vi "ROI entry-Handle ROI change.vi"(7 "Selected ROI":i32[](array[numeric]), 8 "error in (no error)":errorcluster, 9 "Offsets cluster":T1, 11 "ROI management":T2) -> (0 "error out":errorcluster, 2 "No ROI":bool, 3 "Number of ROI":i32)   [LabVIEW 2020]
uses:
  Typedefs/ROI management FG states.ctl
  Typedefs/Offsets cluster.ctl
  ROI Entry screen/Typedefs/Redraw ROI.ctl
  ROI Entry screen/Typedefs/FGV ROI Time Ops.ctl
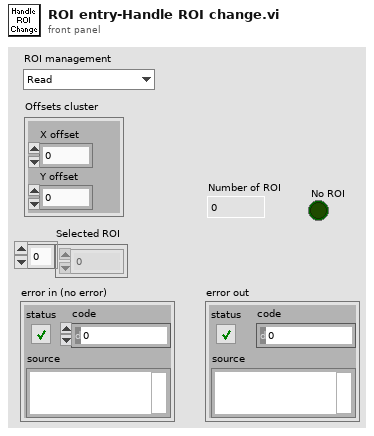
[diagram p1: front panel]
types:
  T1 = typedef "Offsets cluster.ctl" = cluster{"X offset":i8, "Y offset":i8}
  T2 = typedef "ROI management FG states.ctl" = enum16{"Read", "Write", "Write-from dataset", "Clear Last", "Clear All", "Delete ROI", "Update ROIs time", "Reload last ROI set", "Modify ROI Parameters", "Offset all ROI", "Offset visible ROI", "Modify Dwell Time", "Modify Laser Power"}
  T3 = typedef "FGV ROI Time Ops.ctl" = enum16{"Read", "Write Cycle Time", "Write Cycle Rate"}
  T4 = typedef "Redraw ROI.ctl" = enum16{"Redraw All", "Redraw Deselected", "Draw Last", "Redraw Selected"}
  T5 = typedef "ROI parameters data type.ctl" = cluster{"ROI index":dbl, "ROI ID":dbl, "ROI Time (ns)":dbl, "Pixels in ROI":dbl, "X start":dbl, "Y start":dbl, "Z start":dbl, "X stop":dbl, "Y stop":dbl, "Z stop":dbl, "Angle (deg)":dbl, "Composite ID":dbl, "Number of lines":dbl, "Frame Size":dbl, "Zoom":dbl, "Laser Power (%)":dbl, "ROI group ID":dbl, "Resolution":dbl, "Dwell Time per pixel":dbl, "Pixels per miniscan":dbl, "Original FOV (um)":dbl, "Apparent Frame Size":dbl, "Z Plane Idx":i32[], "Z Plane codes":i32[]}
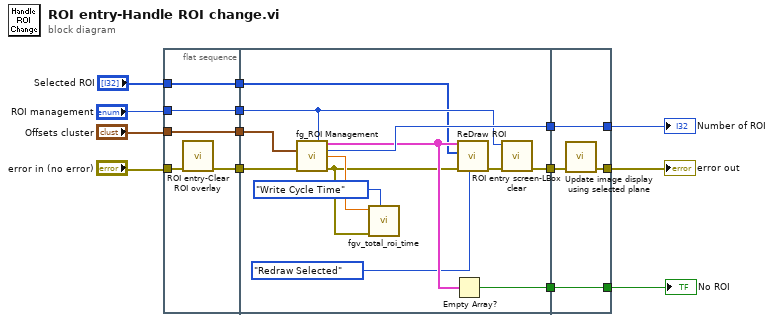
[diagram p0: block diagram]
diagram:
  n1 = flat-sequence {
    tunnel: [w19] -> w14
    tunnel: "error in (no error)" -> [w18]
    tunnel: [w17] -> w10
    tunnel: "ROI management" -> [w17]
    tunnel: "Offsets cluster" -> [w16]
    tunnel: [w16] -> w3
    tunnel: "Selected ROI" -> [w15]
    tunnel: [w15] -> w1
    tunnel: [w26] -> w13
    tunnel: w14 -> [w32]
    tunnel: w10 -> [w25]
    tunnel: [w31] -> w7
    tunnel: [w30] -> w6
    tunnel: w3 -> [w28]
    tunnel: w1 -> [w23]
    tunnel: [w33] -> w11
    tunnel: w13 -> [w34]
    tunnel: [w36] -> w8
    tunnel: w7 -> [w36]
    tunnel: [w35] -> w5
    tunnel: w6 -> [w35]
    frame #0 {
      n2 = call "ROI entry-Clear ROI overlay.vi"("error in (no error)"=w18) -> ("error out"=w19:errorcluster)  [unwired: 9 in, 1 out]
    }
    frame #1 {
      n3 = call "fg_ROI Management.vi"("Function"=w25, "Offsets cluster"=w28, "error in (no error)"=w32) -> ("ROI Setup"=w29:T5[], "Number of ROI"=w31:i32, "Total ROI time"=w22:dbl, "error out"=w21:errorcluster)  [unwired: 6 in, 3 out]
      n4 = call "fgv_total_roi_time.vi"("Op"=FGV_ROI_Time_Ops."Write Cycle Time", "error in (no error)"=w21, "Total cycle time"=w22) -> ()  [unwired: 4 in, 5 out]
      n5 = Empty Array?(array=w29) -> (empty?=w30:bool)
      n6 = call "ReDraw ROI.vi"("Mode (Redraw All)"=Redraw_ROI."Redraw Selected", "error in"=w21, "Selected/Deselected"=w23, "XYZ Coordinates"=w29) -> ("error out"=w27:errorcluster)  [unwired: 7 in]
      n7 = call "ROI entry screen-LBox clear.vi"("error in (no error)"=w27, "Function"=w25) -> ("error out"=w26:errorcluster)  [unwired: 9 in]
    }
    frame #2 {
      n8 = call "Update image display using selected plane.vi"("error in (no error)"=w34) -> ("error out"=w33:errorcluster)  [unwired: 10 in]
    }
  }
  "error out" <- w11
  "Number of ROI" <- w8
  "No ROI" <- w5
